vi "Update Method Accessors.vi"(7 "Library":refnum<vi>, 8 "error in (no error)":errorcluster, 10 "RPC Method Parameters":T1, 11 "Server class in":refnum<vi>) -> (0 "error out":errorcluster, 3 "Server class out":refnum<vi>)   [LabVIEW 2019, in "gRPC Template Creation Utility.lvlib"]
uses:
  gRPC Template Creation Utility.lvlib
  TypeDefs/RPC Method Parameters.ctl
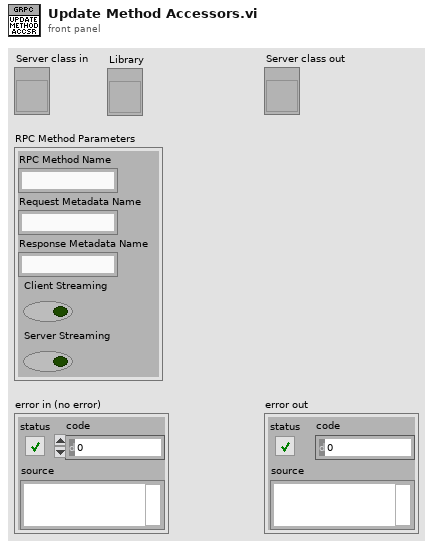
[diagram p1: front panel]
types:
  T1 = typedef "gRPC Template Creation Utility.lvlib/RPC Method Parameters.ctl" = cluster{"RPC Method Name":string, "Request Metadata Name":string, "Response Metadata Name":string, "Client Streaming":bool, "Server Streaming":bool}
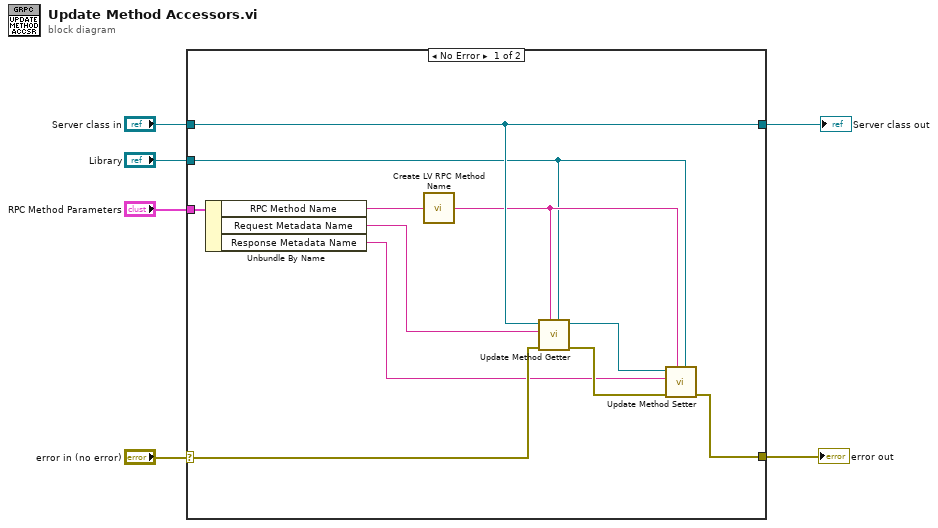
[diagram p0: block diagram]
diagram:
  n1 = case shown="No Error" "error in (no error)" {
    selector: "error in (no error)" -> [w15 w18]
    tunnel: "RPC Method Parameters" -> [w17 _]
    tunnel: "Server class in" -> [w10 w19]
    tunnel: [w10 w19] -> w3
    tunnel: [w11 w18] -> w2
    tunnel: "Library" -> [w7 _]
    frame No Error {
      n2 = Unbundle By Name(w17) -> ("RPC Method Name"=w9:string, "Request Metadata Name"=w16:string, "Response Metadata Name"=w12:string)
      n3 = call "Create LV RPC Method Name.vi"("Proto Parser RPC Method Name in"=w9) -> ("LV RPC Method Name out"=w8:string)
      n4 = call "Update Method Getter.vi"("Library"=w7, "RPC Method Name"=w8, "error in (no error)"=w15, "Request Metadata Name"=w16, "Server class in"=w10) -> ("error out"=w14:errorcluster, "Server class out"=w13:refnum<vi>)  [unwired: 5 in]
      n5 = call "Update Method Setter.vi"("Library"=w7, "RPC Method Name"=w8, "error in (no error)"=w14, "Response Metadata Name"=w12, "Server class in"=w13) -> ("error out"=w11:errorcluster)  [unwired: 5 in, 1 out]
    }
    frame Error {
    }
  }
  "error out" <- w2
  "Server class out" <- w3
